vi "Pass If In 1D Array (SGL).vi"(6 "expected index (optional)":i32=-1, 7 "custom report message (\"\")":string, 8 "error in (no error)":errorcluster, 9 "element":sgl, 10 "1D array":sgl[](array[numeric]), 11 "TestCase in":refnum<class "TestCase.lvclass">) -> (0 "error out":errorcluster, 3 "TestCase out":refnum<class "TestCase.lvclass">)   [LabVIEW 2015, in "VITAC.lvlib"]
doc: "Searches element in 1D SGL array, and returns pass if element is found. If <b>expected index (optional)</b> does not equal to -1, additionally compares found index with expected; and fails if they are not equal."
uses:
  VITAC.lvlib
  <vilib>/addons/_JKI Toolkits/VI Tester/TestCase.llb/TestCase.lvclass
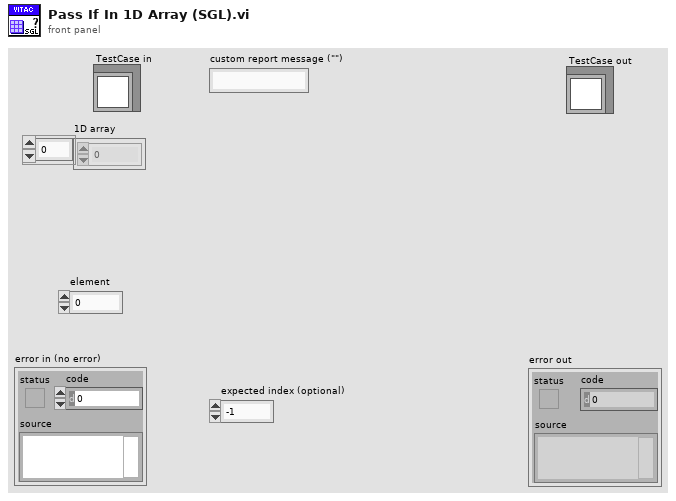
[diagram p1: front panel]
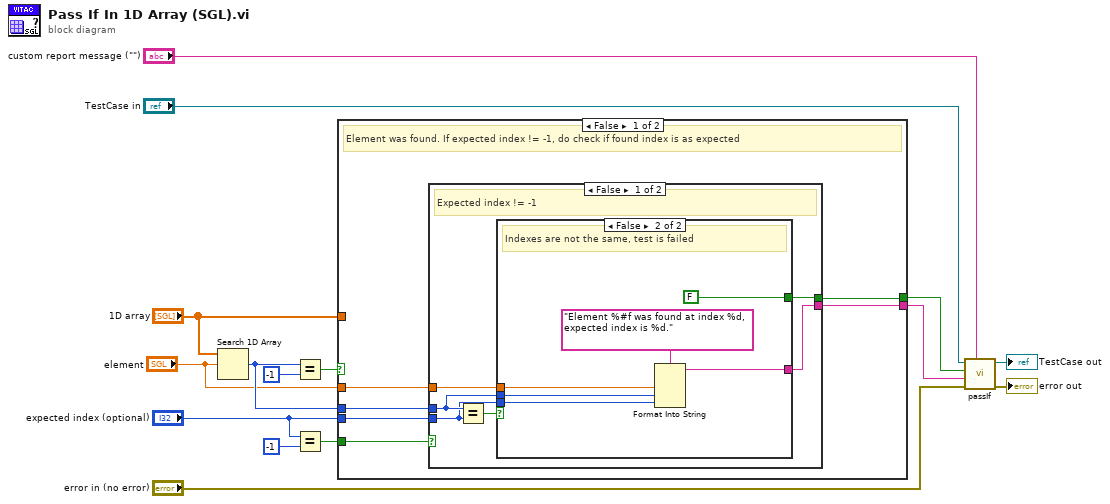
[diagram p0: block diagram]
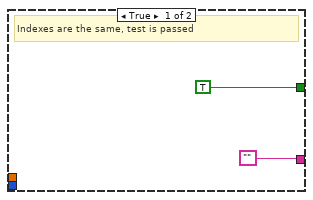
[diagram p2: hidden frame]
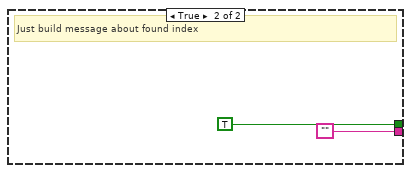
[diagram p3: hidden frame]
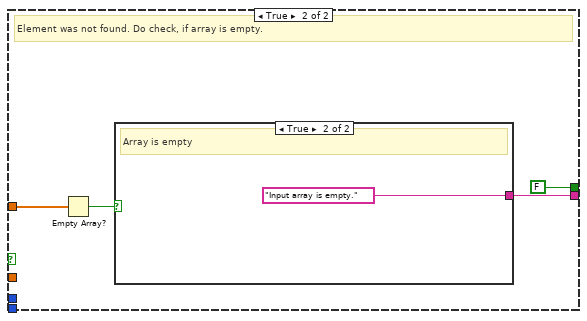
[diagram p4: hidden frame]
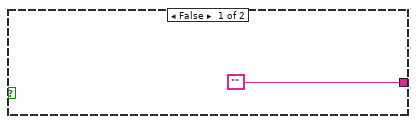
[diagram p5: hidden frame]
diagram:
  n1 = Search 1D Array(1D array="1D array", element="element") -> (index of element=w6:i32)  [unwired: 1 in]
  n2 = Equal?(x=w6, y=-1) -> (x = y?=w9:bool)
  n3 = Equal?(x="expected index (optional)", y=-1) -> (x = y?=w3:bool)
  n4 = case shown="False" w9 {
    tunnel: "expected index (optional)" -> [w16 _]
    tunnel: [w20 FALSE] -> w11
    tunnel: [w17 w39] -> w10
    tunnel: "1D array" -> [_ w41]
    tunnel: w6 -> [w18 _]
    tunnel: w3 -> [w21 _]
    tunnel: "element" -> [w19 _]
    frame False {
      # "Element was found. If expected index != -1, do check if found index is as expected"
      n5 = case shown="False" w21 {
        tunnel: [w23 TRUE] -> w20
        tunnel: w19 -> [w26 _]
        tunnel: w18 -> [w25 _]
        tunnel: [w24 ""] -> w17
        tunnel: w16 -> [w22 _]
        frame False {
          # "Expected index != -1"
          n6 = Equal?(x=w25, y=w22) -> (x = y?=w27:bool)
          n7 = case shown="False" w27 {
            tunnel: w26 -> [_ w34]
            tunnel: w25 -> [_ w33]
            tunnel: ["" w32] -> w24
            tunnel: [TRUE FALSE] -> w23
            tunnel: w22 -> [_ w30]
            frame True {
              # "Indexes are the same, test is passed"
            }
            frame False {
              # "Indexes are not the same, test is failed"
              n8 = Format Into String(format string="Element %#f was found at index %d, expected index is %d.", w34, w33, w30) -> (resulting string=w32:string)  [unwired: 2 in, 1 out]
            }
          }
        }
        frame True {
          # "Just build message about found index"
        }
      }
    }
    frame True {
      # "Element was not found. Do check, if array is empty."
      n9 = Empty Array?(array=w41) -> (empty?=w40:bool)
      n10 = case shown="True" w40 {
        tunnel: ["" "Input array is empty."] -> w39
        frame False {
        }
        frame True {
          # "Array is empty"
        }
      }
    }
  }
  n11 = call-dynamic "passIf.vi"("custom report message (\"\")"="custom report message (\"\")", "error in (no error)"="error in (no error)", "message (\"\")"=w10, "pass"=w11, "TestCase in"="TestCase in") -> ("error out"=→"error out":errorcluster, "TestCase out"=→"TestCase out":refnum<class "TestCase.lvclass">)  [unwired: 5 in]
